vi "DF_prototype_automated.vi"() -> ()   [LabVIEW 2019]
uses:
  Control 3.ctl
  <vilib>/Instr/_visa.llb/VISA Configure Serial Port (Instr).vi
panel:
  out "Elapsed Time/check every 20min":string caption="Elapsed Time Text"
  in  "Flow controller (bar)":T1 step=0.1 format="%#_4g"
  in  "Pump speed (%)":T1 step=0.1 format="%#_4g"
  in  "Pump port":refnum<visa-resource-name>="COM4"
  in  "CB speed (Hz)":T1 step=0.1 format="%#_4g"
  in  "Stop CB":bool
  out "CB cable correctly connected ?":bool
  in  "CB port":refnum<visa-resource-name>="COM12"
  out "error out":errorcluster={"status"=FALSE, "code"=1073676294, "source"="VISA Read in DF_prototype_automated.vi"}
  in  "Stop pump":bool
  out "Pump cable correctly connected ?":bool
  out "Error Out":errorcluster={"status"=FALSE, "code"=1073676294, "source"="VISA Read in DF_prototype_automated.vi"}
  out "Error":string="LabJack Error #1224:  LJME_DEVICE_NOT_OPEN occurred at LJM_eReadAddresses.vi"
  out "Pressure in the foamer (bar)":dbl(graph)
  in  "Stop Foam":bool
  # "FEEDING PUMP"
  # "|\n|\n|\n|\n|\n|\n|\n|\n|\n|\n|\n|\n|\n|\n|\n|\n|\n|\n|\n|\n|\n|\n|\n|\n|\n|\n|\n|\n|"
  # "PRESSURE REGULATOR"
  # "|\n|\n|\n|\n|\n|\n|\n|\n|\n|\n|\n|\n|\n|\n|\n|\n|\n|\n|\n|\n|\n|\n|\n|\n|\n|\n|\n|\n|"
  # "|\n|\n|\n|\n|\n|\n|\n|\n|\n|\n|\n|\n|\n|\n|\n|\n|\n|\n|\n|\n|\n|\n|\n|\n|\n|\n|\n|\n|"
  # "CONVEYER BELT"
  # "|\n|\n|\n|\n|\n|\n|\n|\n|\n|\n|\n|\n|\n|\n|\n|\n|\n|\n|\n|\n|\n|\n|\n|\n|\n|\n|\n|\n|"
  # "0,9 bar is good"
  # "6 Hz is good"
  # "sign -+ change direction"
  # "40% is good"
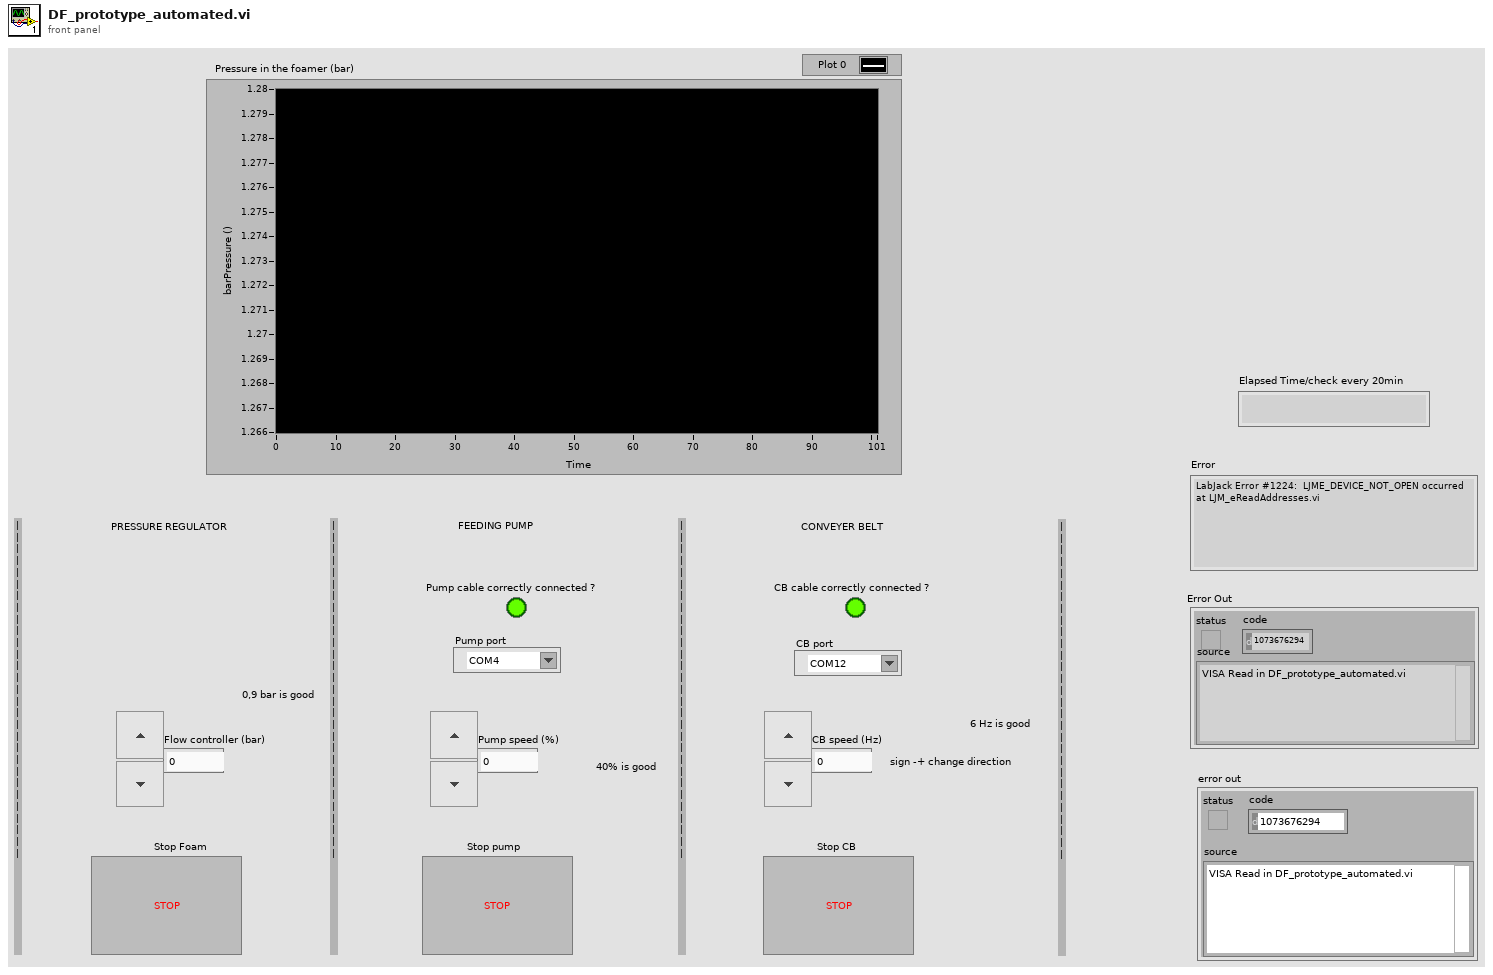
[diagram p1: front panel]
types:
  T1 = typedef "Control 3.ctl" = dbl
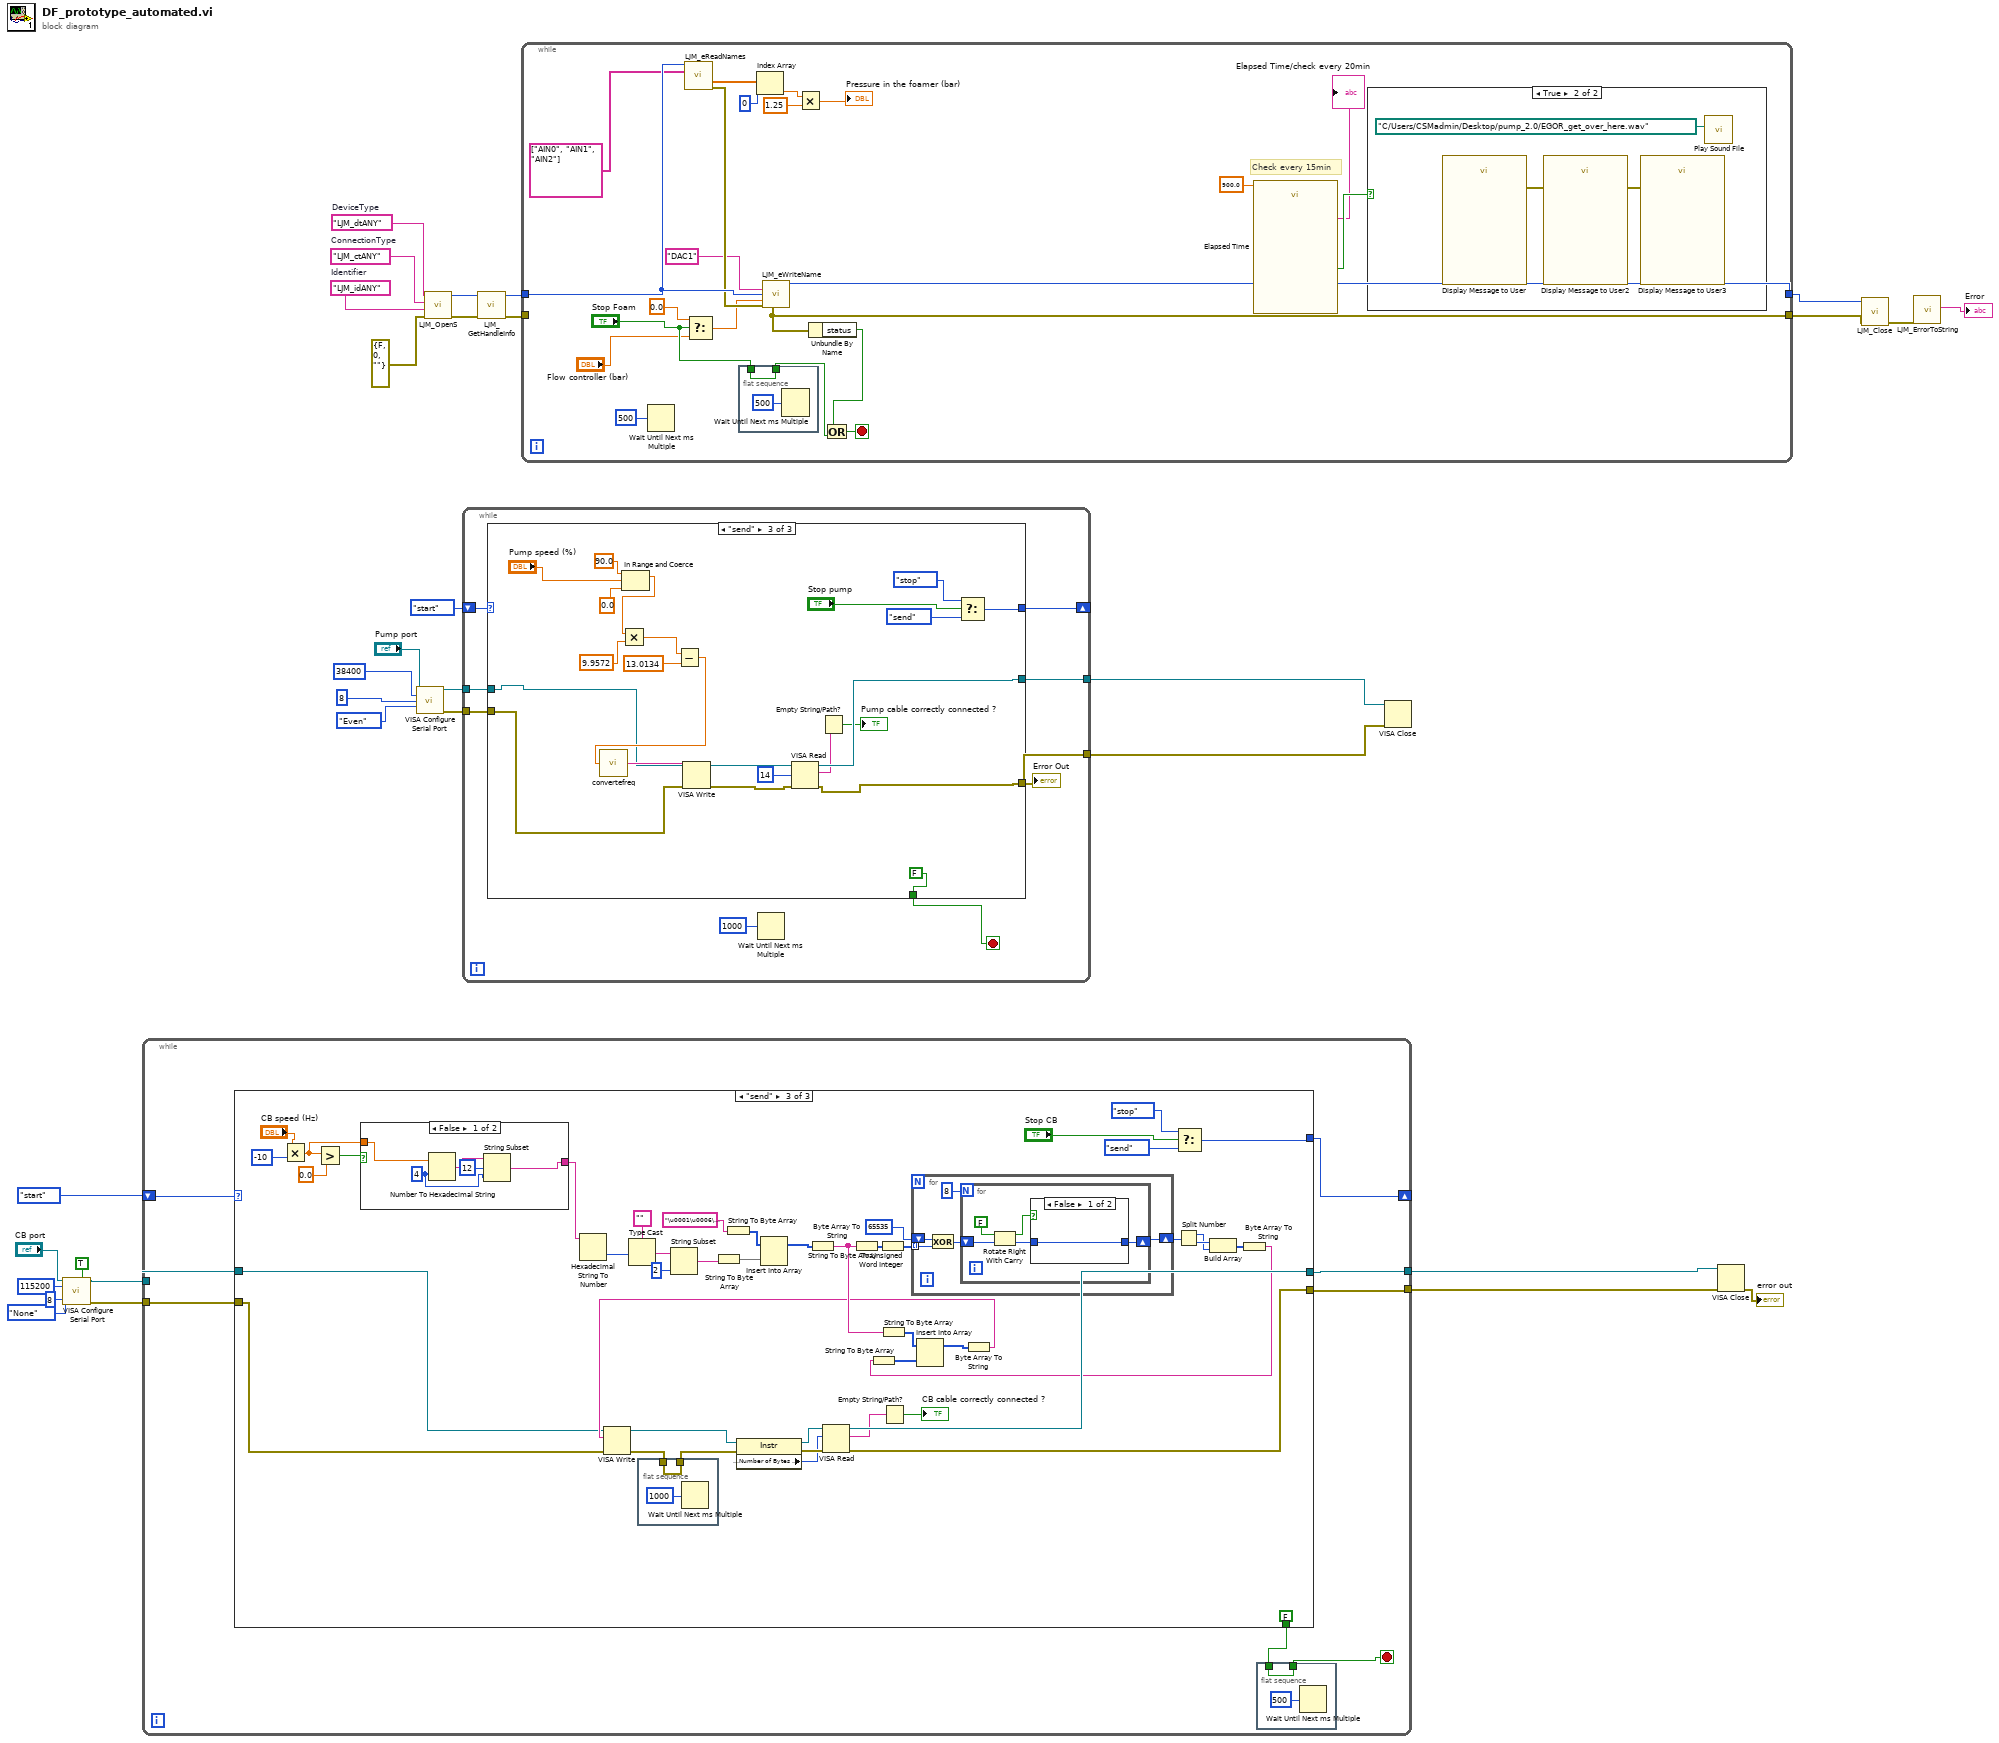
[diagram p0: block diagram]
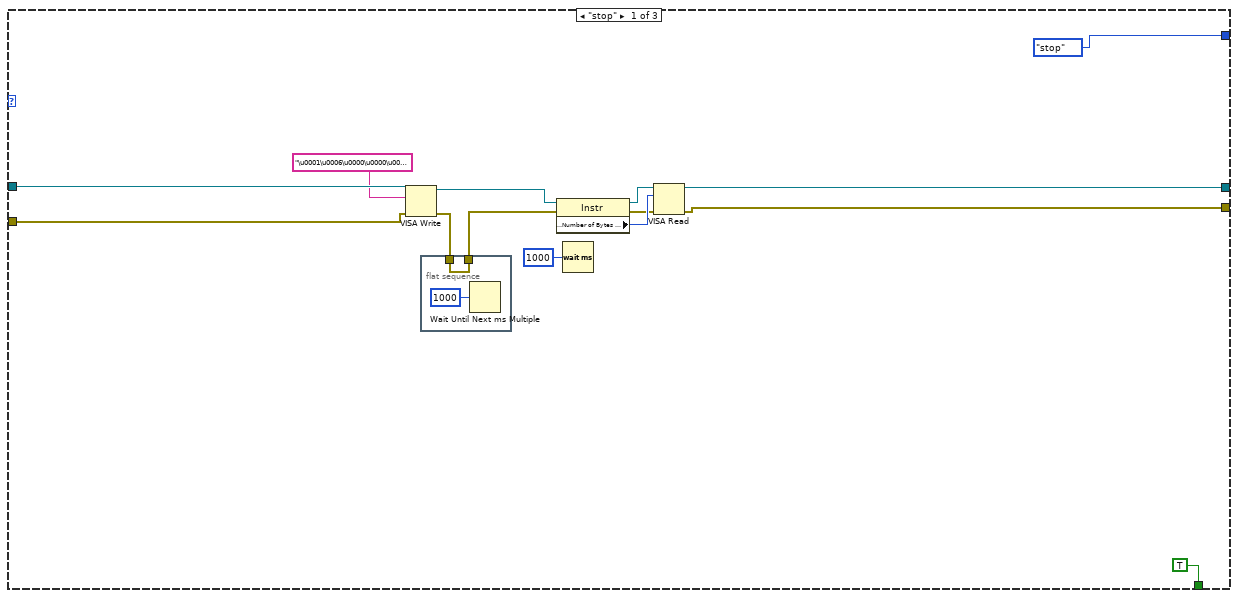
[diagram p2: hidden frame]
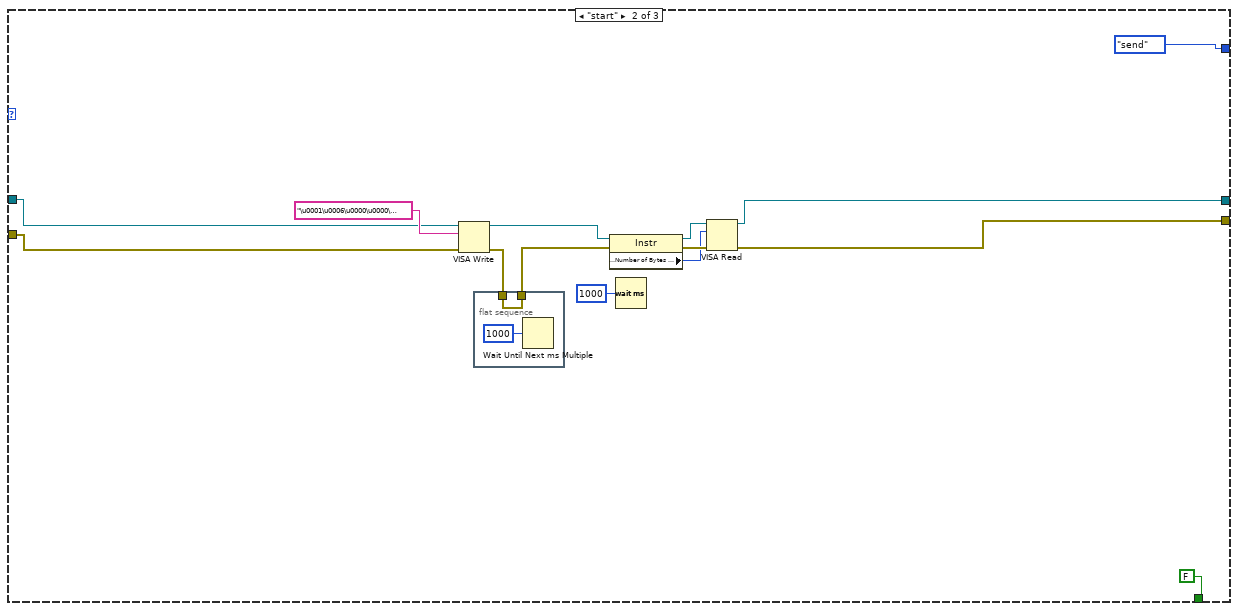
[diagram p3: hidden frame]
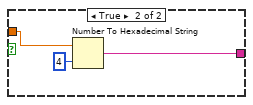
[diagram p4: hidden frame]
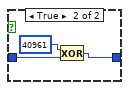
[diagram p5: hidden frame]
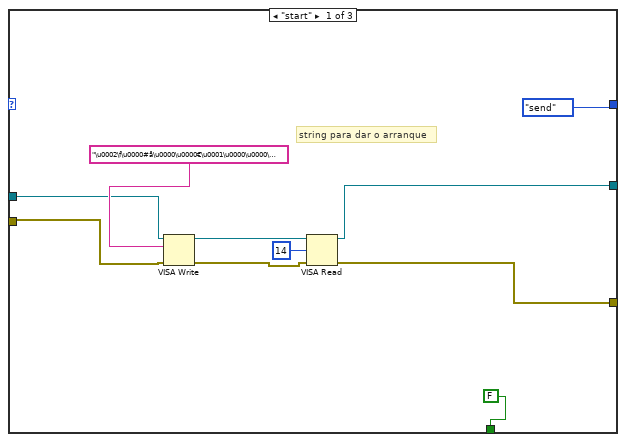
[diagram p6: hidden frame]
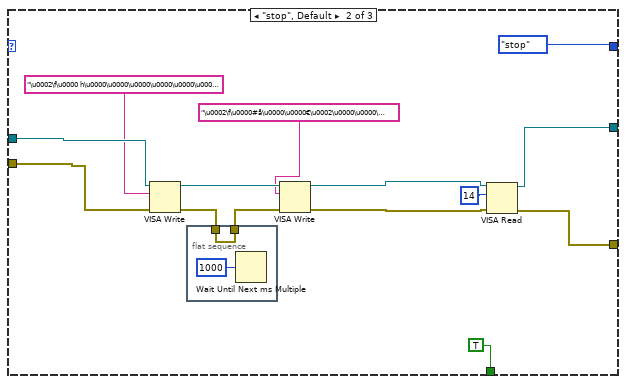
[diagram p7: hidden frame]
diagram:
  w22 = "LJM_idANY"  # Identifier
  w23 = "LJM_ctANY"  # ConnectionType
  w24 = "LJM_dtANY"  # DeviceType
  n1 = call-poly "VISA Configure Serial Port"("VISA resource name"="CB port", "Enable Termination\nChar (T)"=TRUE ("Enable Termination\nChar (T)"), "baud rate (9600)"=u32 115200, "data bits (8)"=u16 8, "parity (0:none)"=enum16{"None", "Odd", "Even", "Mark", "Space"}."None") -> ("VISA resource name out"=w8:refnum<visa-resource-name>, "error out"=w7:errorcluster)  [unwired: 2 in, 7 out]
  n2 = while {
    tunnel: [w37] -> w11
    tunnel: [w38] -> w10
    tunnel: w8 -> [w39]
    tunnel: w7 -> [w40]
    shift-right: [w36] -> _
    shift-left: enum16{"stop", "start", "send"}."start" -> [w35]
    stop <- w33 stop-if-true
    n3 = case shown="\"send\"" w35 {
      tunnel: w39 -> [w52 w64 w89]
      tunnel: w40 -> [w51 w63 w88]
      tunnel: [w49 w61 w112] -> w37
      tunnel: [w50 w62 w113] -> w38
      tunnel: [enum16{"stop", "start", "send"}."stop" enum16{"stop", "start", "send"}."send" w85] -> w36
      tunnel: [TRUE FALSE FALSE] -> w34
      frame "stop" {
        n4 = VISA Write(VISA resource name=w52, write buffer="\u0001\u0006\u0000\u0000\u0000\u0000‰Ê" ("write buffer (\"\")"), error in (no error)=w51) -> (VISA resource name out=w54:refnum<visa-resource-name>, error out=w46:errorcluster)  [unwired: 1 out]
        n5 = flat-sequence {
          tunnel: [w57] -> w45
          tunnel: w46 -> [w57]
          frame #0 {
            n6 = Wait Until Next ms Multiple(millisecond multiple=u32 1000) -> ()  [unwired: 1 out]
          }
        }
        n7 = property on="Property Node" class="Instr"(reference=w54, error in=w45) -> (reference out=w55:refnum<visa-resource-name>, error out=w53:errorcluster, "Serial Settings:Number of Bytes at Serial Port"=w56:u32)
        n8 = Wait (ms)(milliseconds to wait=u32 1000) -> ()  [unwired: 1 out]
        n9 = VISA Read(VISA resource name=w55, byte count=w56, error in (no error)=w53) -> (VISA resource name out=w50:refnum<visa-resource-name>, error out=w49:errorcluster)  [unwired: 2 out]
      }
      frame "start" {
        n10 = VISA Write(VISA resource name=w64, write buffer="\u0001\u0006\u0000\u0000\u0000\u0001H\n" ("write buffer (\"\")"), error in (no error)=w63) -> (VISA resource name out=w69:refnum<visa-resource-name>, error out=w71:errorcluster)  [unwired: 1 out]
        n11 = flat-sequence {
          tunnel: [w73] -> w72
          tunnel: w71 -> [w73]
          frame #0 {
            n12 = Wait Until Next ms Multiple(millisecond multiple=u32 1000) -> ()  [unwired: 1 out]
          }
        }
        n13 = property on="Property Node" class="Instr"(reference=w69, error in=w72) -> (reference out=w68:refnum<visa-resource-name>, error out=w70:errorcluster, "Serial Settings:Number of Bytes at Serial Port"=w67:u32)
        n14 = Wait (ms)(milliseconds to wait=u32 1000) -> ()  [unwired: 1 out]
        n15 = VISA Read(VISA resource name=w68, byte count=w67, error in (no error)=w70) -> (VISA resource name out=w62:refnum<visa-resource-name>, error out=w61:errorcluster)  [unwired: 2 out]
      }
      frame "send" {
        n16 = Multiply(x="CB speed (Hz)", y=-10) -> (x*y=w78:T1)
        n17 = Greater?(x=w78, y=T1 0.0) -> (0:w79:bool)
        n18 = case shown="False" w79 {
          tunnel: w78 -> [w123 w126]
          tunnel: [w122 w125] -> w77
          frame False {
            w121 = i16 4 ("width (-)")
            n19 = Number To Hexadecimal String(1:w121, 2:w123) -> (0:w124:string)
            n20 = String Subset(string=w124, offset (0)=12, length (rest)=w121) -> (substring=w122:string)
          }
          frame True {
            n21 = Number To Hexadecimal String(1:i16 4 ("width (-)"), 2:w126) -> (0:w125:string)
          }
        }
        n22 = Hexadecimal String To Number(string=w77) -> (number=w100:u32)  [unwired: 2 in, 1 out]
        n23 = Type Cast(type="" ("write buffer (\"\")"), x=w100) -> (*(type *) &x=w98:string)
        n24 = flat-sequence {
          tunnel: [w142] -> w115
          tunnel: w114 -> [w142]
          frame #0 {
            n25 = Wait Until Next ms Multiple(millisecond multiple=u32 1000) -> ()  [unwired: 1 out]
          }
        }
        n26 = String Subset(string=w98, offset (0)=2) -> (substring=w96:string)  [unwired: 1 in]
        n27 = String To Byte Array(string=w96) -> (unsigned byte array=w103:u8[])
        n28 = String To Byte Array(string="\u0001\u0006\u0000\u0001" ("write buffer (\"\")")) -> (unsigned byte array=w104:u8[])
        n29 = Insert Into Array(array=w104, new element=w103) -> (w102:u8[])  [unwired: 1 in]
        n30 = Byte Array To String(unsigned byte array=w102) -> (string=w92:string)
        n31 = String To Byte Array(string=w92) -> (unsigned byte array=w109:u8[])
        n32 = To Unsigned Word Integer(number=w109) -> (unsigned 16bit integer=w108:u16[])
        n33 = String To Byte Array(string=w92) -> (unsigned byte array=w95:u8[])
        n34 = for {
          shift-right: [w129] -> w110
          shift-left: u16 65535 -> [w130]
          tunnel: w108 -> [w128] mode=indexing
          n35 = Exclusive Or(1:w128, 2:w130) -> (0:w131:u16)
          n36 = for {
            N: 8 -> [_]
            shift-right: [w136] -> w129
            shift-left: w131 -> [w135]
            n37 = Rotate Right With Carry(2:w135, 3:FALSE ("Übertrag")) -> (0:w137:u16, 1:w134:bool)
            n38 = case shown="False" w134 {
              tunnel: w137 -> [w138 w140]
              tunnel: [w138 w139] -> w136
              frame False {
              }
              frame True {
                n39 = Exclusive Or(1:w140, 2:u16 40961) -> (0:w139:u16)
              }
            }
          }
        }
        n40 = Select(t=enum16{"stop", "start", "send"}."stop", s="Stop CB", f=enum16{"stop", "start", "send"}."send") -> (s? t:f=w85:enum16{"stop", "start", "send"})
        n41 = Split Number(x=w110) -> (hi(x)=w106:u8, lo(x)=w107:u8)
        n42 = Build Array(w107, w106) -> (w105:u8[])
        n43 = Byte Array To String(unsigned byte array=w105) -> (string=w91:string)
        n44 = String To Byte Array(string=w91) -> (unsigned byte array=w94:u8[])
        n45 = Insert Into Array(array=w95, new element=w94) -> (w93:u8[])  [unwired: 1 in]
        n46 = Byte Array To String(unsigned byte array=w93) -> (string=w90:string)
        n47 = VISA Write(VISA resource name=w89, write buffer=w90, error in (no error)=w88) -> (VISA resource name out=w118:refnum<visa-resource-name>, error out=w114:errorcluster)  [unwired: 1 out]
        n48 = property on="Property Node" class="Instr"(reference=w118, error in=w115) -> (reference out=w117:refnum<visa-resource-name>, error out=w119:errorcluster, "Serial Settings:Number of Bytes at Serial Port"=w116:u32)
        n49 = VISA Read(VISA resource name=w117, byte count=w116, error in (no error)=w119) -> (VISA resource name out=w113:refnum<visa-resource-name>, read buffer=w76:string, error out=w112:errorcluster)  [unwired: 1 out]
        n50 = Empty String/Path?(string/path=w76) -> (empty?=→"CB cable correctly connected ?":bool)
      }
    }
    n51 = flat-sequence {
      tunnel: w34 -> [w41]
      tunnel: [w41] -> w33
      frame #0 {
        n52 = Wait Until Next ms Multiple(millisecond multiple=u32 500) -> ()  [unwired: 1 out]
      }
    }
  }
  n53 = call-poly "VISA Configure Serial Port"("VISA resource name"="Pump port", "baud rate (9600)"=u32 38400, "data bits (8)"=u16 8, "parity (0:none)"=enum16{"None", "Odd", "Even", "Mark", "Space"}."Even") -> ("VISA resource name out"=w19:refnum<visa-resource-name>, "error out"=w18:errorcluster)  [unwired: 10 in]
  n54 = call "LJM_OpenS.vi"("error in"=errorcluster {"status"=FALSE, "code"=0, "source"=""} ("error in (no error)"), "Identifier"=w22, "ConnectionType"=w23, "DeviceType"=w24) -> ("error out"=w31:errorcluster, "Handle"=w30:i32)  [unwired: 6 in]
  n55 = while {
    tunnel: w19 -> [w150]
    tunnel: w18 -> [w151]
    tunnel: [w149] -> w17
    tunnel: [w148] -> w16
    shift-right: [w146] -> _
    shift-left: enum16{"stop", "start", "send"}."start" -> [w147]
    stop <- w145 stop-if-true
    n56 = case shown="\"send\"" w147 {
      tunnel: w150 -> [w156 w175 w190]
      tunnel: w151 -> [w157 w174 w189]
      tunnel: [w160 w173 w187] -> w148
      tunnel: [w155 w171 w188] -> w149
      tunnel: [enum16{"stop", "start", "send"}."send" enum16{"stop", "start", "send"}."stop" w183] -> w146
      tunnel: [FALSE TRUE FALSE] -> w145
      frame "start" {
        # "string para dar o arranque"
        n57 = VISA Write(VISA resource name=w156, write buffer="\u0002\f\u0000#å\u0000\u0000€\u0001\u0000\u0000\u0000\u0000I" ("write buffer (\"\")"), error in (no error)=w157) -> (VISA resource name out=w159:refnum<visa-resource-name>, error out=w153:errorcluster)  [unwired: 1 out]
        n58 = VISA Read(VISA resource name=w159, byte count=u32 14 ("Bytes to Read"), error in (no error)=w153) -> (VISA resource name out=w155:refnum<visa-resource-name>, error out=w160:errorcluster)  [unwired: 2 out]
      }
      frame "stop", Default {
        n59 = VISA Write(VISA resource name=w175, write buffer="\u0002\f\u0000 h\u0000\u0000\u0000\u0000\u0000\u0000\u0000\u0000F" ("write buffer (\"\")"), error in (no error)=w174) -> (VISA resource name out=w166:refnum<visa-resource-name>, error out=w168:errorcluster)  [unwired: 1 out]
        n60 = flat-sequence {
          tunnel: [w176] -> w167
          tunnel: w168 -> [w176]
          frame #0 {
            n61 = Wait Until Next ms Multiple(millisecond multiple=u32 1000) -> ()  [unwired: 1 out]
          }
        }
        n62 = VISA Write(VISA resource name=w166, write buffer="\u0002\f\u0000#å\u0000\u0000€\u0002\u0000\u0000\u0000\u0000J" ("write buffer (\"\")"), error in (no error)=w167) -> (VISA resource name out=w165:refnum<visa-resource-name>, error out=w162:errorcluster)  [unwired: 1 out]
        n63 = VISA Read(VISA resource name=w165, byte count=u32 14 ("Bytes to Read"), error in (no error)=w162) -> (VISA resource name out=w171:refnum<visa-resource-name>, error out=w173:errorcluster)  [unwired: 2 out]
      }
      frame "send" {
        n64 = In Range and Coerce(upper limit=90.0, x="Pump speed (%)", lower limit=0.0) -> (coerced(x)=w192:T1)  [unwired: 1 out]
        n65 = Multiply(x=w192, y=9.9572) -> (x*y=w195:T1)
        n66 = Subtract(x=w195, y=13.0134) -> (x-y=w194:T1)
        n67 = call "convertefreq.vi"("Numeric"=w194) -> ("string"=w198:string)
        n68 = VISA Write(VISA resource name=w190, write buffer=w198, error in (no error)=w189) -> (VISA resource name out=w200:refnum<visa-resource-name>, error out=w178:errorcluster)  [unwired: 1 out]
        n69 = VISA Read(VISA resource name=w200, byte count=u32 14 ("Bytes to Read"), error in (no error)=w178) -> (VISA resource name out=w188:refnum<visa-resource-name>, read buffer=w180:string, error out=w187:errorcluster)  [unwired: 1 out]
        n70 = Empty String/Path?(string/path=w180) -> (empty?=→"Pump cable correctly connected ?":bool)
        n71 = Select(t=enum16{"stop", "start", "send"}."stop", s="Stop pump", f=enum16{"stop", "start", "send"}."send") -> (s? t:f=w183:enum16{"stop", "start", "send"})
      }
    }
    "Error Out" <- w148
    n72 = Wait Until Next ms Multiple(millisecond multiple=u32 1000) -> ()  [unwired: 1 out]
  }
  n73 = call "LJM_GetHandleInfo.vi"("error in"=w31, "Handle In"=w30) -> ("error out"=w25:errorcluster, "Handle Out"=w26:i32)  [unwired: 2 in, 6 out]
  n74 = while {
    tunnel: w25 -> [_]
    tunnel: [w219] -> w28
    tunnel: w26 -> [w217]
    tunnel: [w220] -> w27
    stop <- w222 stop-if-true
    # "Check every 15min"
    n75 = Wait Until Next ms Multiple(millisecond multiple=u32 500) -> ()  [unwired: 1 out]
    n76 = call "LJM_eReadNames.vi"("Handle In"=w217, "aNames"=string[] ["AIN0", "AIN1", "AIN2"]) -> ("aValuesOut"=w215:dbl[], "error out"=w216:errorcluster)  [unwired: 10 in, 2 out]
    n77 = Select(t=0.0, s="Stop Foam", f="Flow controller (bar)") -> (s? t:f=w207:T1)
    n78 = flat-sequence {
      tunnel: "Stop Foam" -> [w226]
      tunnel: [w226] -> w205
      frame #0 {
        n79 = Wait Until Next ms Multiple(millisecond multiple=u32 500) -> ()  [unwired: 1 out]
      }
    }
    n80 = Index Array(array=w215, index=0) -> (element=w213:dbl)
    n81 = call "LJM_eWriteName.vi"("Handle In"=w217, "Name"="DAC1", "Value"=w207, "error in"=w216) -> ("Handle Out"=w220:i32, "error out"=w219:errorcluster)  [unwired: 10 in]
    n82 = Multiply(x=w213, y=1.25) -> (x*y=→"Pressure in the foamer (bar)":dbl)
    n83 = Unbundle By Name(w219) -> ("status"=w221:bool)
    n84 = Or(x=w221, y=w205) -> (x .or. y?=w222:bool)
    n85 = call "Elapsed Time"("Time Target (s)"=900.0) -> ("Time has Elapsed"=w202:bool, "Elapsed Time Text"=→"Elapsed Time/check every 20min":string)  [unwired: 11 in, 6 out]
    n86 = case shown="True" w202 {
      frame False {
      }
      frame True {
        n87 = call "Display Message to User"() -> ("error out"=w224:errorcluster)  [unwired: 10 in, 1 out]
        n88 = call "Display Message to User2"("error in (no error)"=w224) -> ("error out"=w225:errorcluster)  [unwired: 9 in, 1 out]
        n89 = call "Display Message to User3"("error in (no error)"=w225) -> ()  [unwired: 9 in, 2 out]
        n90 = call <vilib>:"Play Sound File.vi"("path"=path "C:/Users/CSMadmin/Desktop/pump_2.0/EGOR_get_over_here.wav") -> ()  [unwired: 9 in, 2 out]
      }
    }
  }
  n91 = VISA Close(VISA resource name=w17, error in (no error)=w16) -> ()  [unwired: 1 out]
  n92 = VISA Close(VISA resource name=w10, error in (no error)=w11) -> (error out=→"error out":errorcluster)
  n93 = call "LJM_Close.vi"("error in"=w28, "Handle"=w27) -> ("error out"=w29:errorcluster)  [unwired: 9 in]
  n94 = call "LJM_ErrorToString.vi"("error in"=w29) -> ("String"=→"Error":string)  [unwired: 10 in]
